vi "IMAQ FPGA Camera Link Acquisition State Machine.vi"(8 "Enables":T2, 9 "Cancel Acq":bool, 10 "Acquire":bool, 11 "Acquisition Settings":T3) -> (0 "Output Valid":bool, 1 "Frame Valid":bool, 2 "Line Valid":bool, 3 "Acquisition Status":T1, 5 "Reset":bool)   [LabVIEW 2017]
doc: "The Acquisition State Machine VI monitors the Camera Link enable signals to determine when pixel data should be captured and when it should be ignored, as indicated by the <B>Output Valid</B>, <B>Frame Valid</B>, and <B>Line Valid</B> outputs. The VI supports finite and continuous acquisitions for both area and line scan cameras. This VI is intended to run within a single-cycle timed loop.\n\nNote that the outputs are delayed by two clock cycles relative to the inputs. Also, this VI does not support cameras that change FVAL while LVAL is asserted. However, FVAL and LVAL are allowed to change at the same time. Open the VI for more documentation."
uses:
  <vilib>/visionFPGA/Basics/Camera Link Acquisition/Controls/IMAQ FPGA Camera Link Acquisition State.ctl
panel:
  # "Refer to the Context Help for a\ndescription of the controls and\nindicators of this VI."
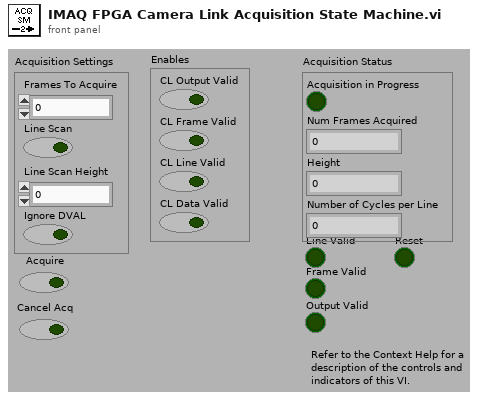
[diagram p1: front panel]
types:
  T1 = cluster{"Acquisition in Progress":bool, "Num Frames Acquired":u32, "Height":u32, "Number of Cycles per Line":u32}
  T2 = cluster{"CL Output Valid":bool, "CL Frame Valid":bool, "CL Line Valid":bool, "CL Data Valid":bool}
  T3 = cluster{"Frames To Acquire":u32, "Line Scan":bool, "Line Scan Height":u32, "Ignore DVAL":bool}
  T4 = typedef "IMAQ FPGA Camera Link Acquisition State.ctl" = enum16{"Idle", "WaitForBlanking", "WaitForStartOfFrame", "WaitForEndOfFrame", "WaitForLastTransition"}
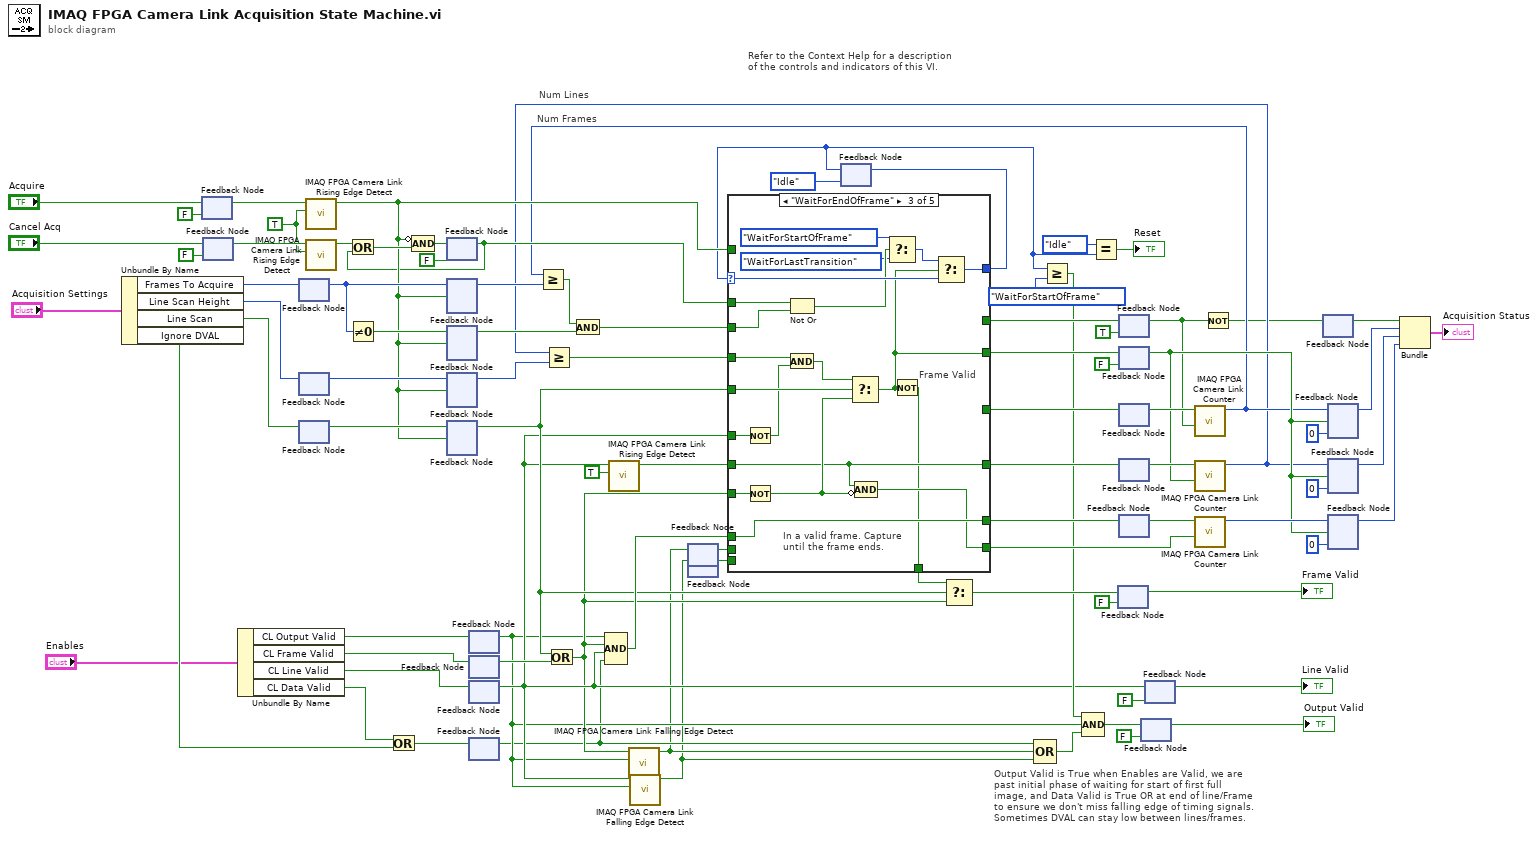
[diagram p0: block diagram]
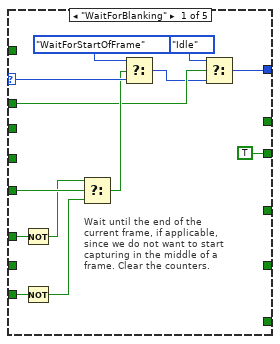
[diagram p2: hidden frame]
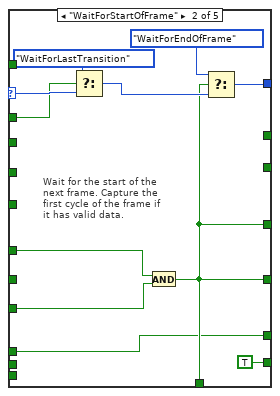
[diagram p3: hidden frame]
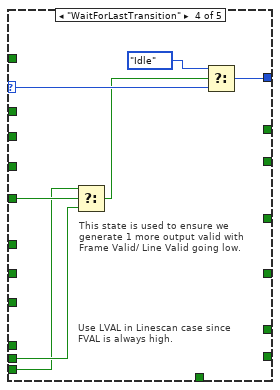
[diagram p4: hidden frame]
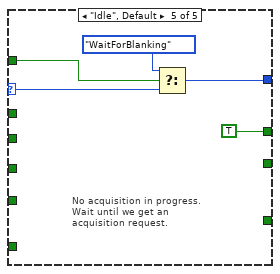
[diagram p5: hidden frame]
diagram:
  w22 = TRUE ("Input Valid")
  # "Num Lines"
  # "Num Frames"
  # "Output Valid is True when Enables are Valid, we are past initial phase of waiting for start of first full image, and Data Valid is True OR at end of line/Frame to ensure we don't miss falling edge of timing signals. Sometimes DVAL can stay low between lines/frames."
  # "Refer to the Context Help for a description\nof the controls and indicators of this VI."
  n1 = Unbundle By Name("Acquisition Settings") -> ("Frames To Acquire"=w37:u32, "Line Scan Height"=w36:u32, "Line Scan"=w35:bool, "Ignore DVAL"=w34:bool)
  n2 = feedback #1(FALSE ("Acquire")) -> (w28:bool)
  n3 = feedback-in #1("Acquire") -> ()
  n4 = feedback #2(FALSE ("Cancel Acq")) -> (w23:bool)
  n5 = feedback-in #2("Cancel Acq") -> ()
  n6 = Unbundle By Name("Enables") -> ("CL Output Valid"=w32:bool, "CL Frame Valid"=w31:bool, "CL Line Valid"=w30:bool, "CL Data Valid"=w29:bool)
  n7 = feedback #3() -> (w76:u32)  [unwired: 1 in]
  n8 = feedback-in #3(w37) -> ()
  n9 = feedback #4() -> (w69:u32)  [unwired: 1 in]
  n10 = feedback-in #4(w36) -> ()
  n11 = feedback #5() -> (w68:bool)  [unwired: 1 in]
  n12 = feedback-in #5(w35) -> ()
  n13 = call <vilib>:"IMAQ FPGA Camera Link Rising Edge Detect.vi"("Input Valid"=w22, "Input"=w28) -> ("Rising Edge"=w27:bool)  [unwired: 9 in]
  n14 = call <vilib>:"IMAQ FPGA Camera Link Rising Edge Detect.vi"("Input Valid"=w22, "Input"=w23) -> ("Rising Edge"=w21:bool)  [unwired: 9 in]
  n15 = Not Equal To 0?(x=w76) -> (x != 0?=w85:bool)
  n16 = Or(x=w29, y=w34) -> (x .or. y?=w39:bool)
  n17 = feedback #6(FALSE) -> (w24:bool)
  n18 = Or(x=w21, y=w24) -> (x .or. y?=w72:bool)
  n19 = Compound Arithmetic op=AND(invert w27, w72) -> (w71:bool)
  n20 = feedback-in #6(w71) -> ()
  n21 = feedback #7() -> (w82:u32)  [unwired: 1 in]
  n22 = feedback-in #7(w76, w27) -> ()
  n23 = feedback #8() -> (w83:bool)  [unwired: 1 in]
  n24 = feedback-in #8(w85, w27) -> ()
  n25 = feedback #9() -> (w67:u32)  [unwired: 1 in]
  n26 = feedback-in #9(w69, w27) -> ()
  n27 = feedback #10() -> (w54:bool)  [unwired: 1 in]
  n28 = feedback-in #10(w68, w27) -> ()
  n29 = feedback #11() -> (w16:bool)  [unwired: 1 in]
  n30 = feedback-in #11(w32) -> ()
  n31 = feedback #12() -> (w48:bool)  [unwired: 1 in]
  n32 = feedback-in #12(w31) -> ()
  n33 = feedback #13() -> (w44:bool)  [unwired: 1 in]
  n34 = feedback-in #13(w30) -> ()
  n35 = feedback #14() -> (w15:bool)  [unwired: 1 in]
  n36 = feedback-in #14(w39) -> ()
  n37 = Or(x=w54, y=w48) -> (x .or. y?=w43:bool)
  n38 = Compound Arithmetic op=AND(w16, w43, w44, w15) -> (w73:bool)
  n39 = call <vilib>:"IMAQ FPGA Camera Link Rising Edge Detect.vi"("Input Valid"=TRUE, "Input"=w44) -> ("Rising Edge"=w70:bool)  [unwired: 9 in]
  n40 = call <vilib>:"IMAQ FPGA Camera Link Falling Edge Detect.vi"("Input Valid"=w16, "Input"=w43) -> ("Falling Edge"=w14:bool)  [unwired: 9 in]
  n41 = call <vilib>:"IMAQ FPGA Camera Link Falling Edge Detect.vi"("Input Valid"=w16, "Input"=w44) -> ("Falling Edge"=w12:bool)  [unwired: 9 in]
  n42 = feedback #15() -> (w13:bool)  [unwired: 1 in]
  n43 = feedback-in #15(w14) -> ()
  n44 = feedback #16() -> (w11:bool)  [unwired: 1 in]
  n45 = feedback-in #16(w12) -> ()
  n46 = feedback #17(IMAQ_FPGA_Camera_Link_Acquisition_State."Idle" ("Enum")) -> (w17:T4)
  n47 = Compound Arithmetic op=OR(w15, w14, w12) -> (w45:bool)
  n48 = Greater Or Equal?(x=w17, y=IMAQ_FPGA_Camera_Link_Acquisition_State."WaitForStartOfFrame") -> (x >= y?=w46:bool)
  n49 = Compound Arithmetic op=AND(w46, w16, w45) -> (w47:bool)
  n50 = Equal?(x=IMAQ_FPGA_Camera_Link_Acquisition_State."Idle", y=w17) -> (x = y?=→"Reset":bool)
  n51 = feedback #18(FALSE) -> (→"Frame Valid":bool)
  n52 = feedback #19(TRUE) -> (w7:bool)
  n53 = feedback #20(FALSE) -> (w59:bool)
  n54 = feedback #21() -> (w87:bool)  [unwired: 1 in]
  n55 = feedback #22() -> (w88:bool)  [unwired: 1 in]
  n56 = feedback #23() -> (w79:bool)  [unwired: 1 in]
  n57 = feedback #24(FALSE) -> (→"Output Valid":bool)
  n58 = feedback-in #24(w47) -> ()
  n59 = feedback-in #25(w44) -> ()
  n60 = feedback #25(FALSE) -> (→"Line Valid":bool)
  n61 = call <vilib>:"IMAQ FPGA Camera Link Counter.vi"("Restart?"=w7, "Increment?"=w87) -> ("Count"=w10:u32)  [unwired: 9 in]
  n62 = Greater Or Equal?(x=w10, y=w82) -> (x >= y?=w84:bool)
  n63 = And(x=w84, y=w83) -> (x .and. y?=w41:bool)
  n64 = call <vilib>:"IMAQ FPGA Camera Link Counter.vi"("Restart?"=w59, "Increment?"=w88) -> ("Count"=w9:u32)  [unwired: 9 in]
  n65 = Greater Or Equal?(x=w9, y=w67) -> (x >= y?=w58:bool)
  n66 = case shown="\"WaitForEndOfFrame\"" w17 {
    selector: w17 -> [w102 w113 w132 w140 w144]
    tunnel: [w95 w110 w133 w139 w145] -> w18
    tunnel: w27 -> [_ _ _ _ w143]
    tunnel: w43 -> [w100 w107 w122 _ _]
    tunnel: [_ w106 w119 _ _] -> w89
    tunnel: [_ w106 _ _ _] -> w86
    tunnel: [TRUE _ w118 _ _] -> w61
    tunnel: w41 -> [_ _ w124 _ _]
    tunnel: [_ _ _ _ TRUE] -> w81
    tunnel: [_ w105 w131 _ _] -> w78
    tunnel: w73 -> [_ w105 w131 _ _]
    tunnel: [_ TRUE w121 _ _] -> w77
    tunnel: w70 -> [_ _ w119 _ _]
    tunnel: w58 -> [_ _ w126 _ _]
    tunnel: w54 -> [w101 _ w129 w137 _]
    tunnel: w24 -> [w97 w109 w125 _ _]
    tunnel: w44 -> [w94 w108 w116 _ _]
    tunnel: [_ w106 w117 _ _] -> w53
    tunnel: w13 -> [_ _ _ w135 _]
    tunnel: w11 -> [_ _ _ w134 _]
    frame "WaitForBlanking" {
      # "Wait until the end of the\ncurrent frame, if applicable,\nsince we do not want to start capturing in the middle of a frame. Clear the counters."
      n67 = Not(x=w94) -> (.not. x?=w93:bool)
      n68 = Not(x=w100) -> (.not. x?=w98:bool)
      n69 = Select(t=w93, s=w101, f=w98) -> (s? t:f=w99:bool)
      n70 = Select(t=IMAQ_FPGA_Camera_Link_Acquisition_State."WaitForStartOfFrame" ("Enum"), s=w99, f=w102) -> (s? t:f=w96:T4)
      n71 = Select(t=IMAQ_FPGA_Camera_Link_Acquisition_State."Idle" ("Enum"), s=w97, f=w96) -> (s? t:f=w95:T4)
    }
    frame "WaitForStartOfFrame" {
      # "Wait for the start of the\nnext frame. Capture the\nfirst cycle of the frame if\nit has valid data."
      n72 = Select(t=IMAQ_FPGA_Camera_Link_Acquisition_State."WaitForLastTransition" ("Enum"), s=w109, f=w113) -> (s? t:f=w111:T4)
      n73 = And(x=w108, y=w107) -> (x .and. y?=w106:bool)
      n74 = Select(t=IMAQ_FPGA_Camera_Link_Acquisition_State."WaitForEndOfFrame" ("Enum"), s=w106, f=w111) -> (s? t:f=w110:T4)
    }
    frame "WaitForEndOfFrame" {
      # "Frame Valid"
      # "In a valid frame. Capture\nuntil the frame ends."
      n75 = Not(x=w116) -> (.not. x?=w128:bool)
      n76 = Not(x=w122) -> (.not. x?=w120:bool)
      n77 = Not Or(1:w124, 2:w125) -> (0:w123:bool)
      n78 = And(x=w126, y=w128) -> (x .and. y?=w127:bool)
      n79 = Select(t=w127, s=w129, f=w120) -> (s? t:f=w118:bool)
      n80 = Compound Arithmetic op=AND(w119, invert w120) -> (w121:bool)
      n81 = Select(t=IMAQ_FPGA_Camera_Link_Acquisition_State."WaitForStartOfFrame" ("Enum"), s=w123, f=IMAQ_FPGA_Camera_Link_Acquisition_State."WaitForLastTransition") -> (s? t:f=w130:T4)
      n82 = Not(x=w118) -> (.not. x?=w117:bool)
      n83 = Select(t=w130, s=w118, f=w132) -> (s? t:f=w133:T4)
    }
    frame "WaitForLastTransition" {
      # "This state is used to ensure we generate 1 more output valid with Frame Valid/ Line Valid going low."
      # "Use LVAL in Linescan case since FVAL is always high."
      n84 = Select(t=w134, s=w137, f=w135) -> (s? t:f=w136:bool)
      n85 = Select(t=IMAQ_FPGA_Camera_Link_Acquisition_State."Idle", s=w136, f=w140) -> (s? t:f=w139:T4)
    }
    frame "Idle", Default {
      # "No acquisition in progress.\nWait until we get an\nacquisition request."
      n86 = Select(t=IMAQ_FPGA_Camera_Link_Acquisition_State."WaitForBlanking", s=w143, f=w144) -> (s? t:f=w145:T4)
    }
  }
  n87 = feedback-in #17(w18) -> ()
  n88 = Select(t=w53, s=w54, f=w43) -> (s? t:f=w52:bool)
  n89 = feedback-in #18(w52) -> ()
  n90 = feedback-in #19(w81) -> ()
  n91 = feedback-in #20(w61) -> ()
  n92 = feedback-in #21(w86) -> ()
  n93 = feedback-in #22(w89) -> ()
  n94 = feedback-in #23(w78) -> ()
  n95 = call <vilib>:"IMAQ FPGA Camera Link Counter.vi"("Restart?"=w77, "Increment?"=w79) -> ("Count"=w80:u32)  [unwired: 9 in]
  n96 = Not(x=w7) -> (.not. x?=w6:bool)
  n97 = feedback #26() -> (w5:bool)  [unwired: 1 in]
  n98 = feedback-in #26(w6) -> ()
  n99 = feedback #27(u32 0 ("Count")) -> (w4:u32)
  n100 = feedback-in #27(w10, w59) -> ()
  n101 = feedback #28(u32 0) -> (w3:u32)
  n102 = feedback-in #28(w9, w59) -> ()
  n103 = feedback #29(u32 0 ("Count")) -> (w2:u32)
  n104 = feedback-in #29(w80, w59) -> ()
  n105 = Bundle(w5, "Count"=w4, w3, "Count"=w2) -> (→"Acquisition Status":cluster{bool, "Count":u32, u32, "Count":u32})  [unwired: 1 in]
